vi "set_distance.vi"(3 "细分":u16=40000, 4 "速度(r/min)":u16, 5 "移动距离(mm)":dbl=1.0 caption="元素") -> (0 "指令":string, 1 "圈数":i32, 2 "脉冲数":i32)   [LabVIEW 2018]
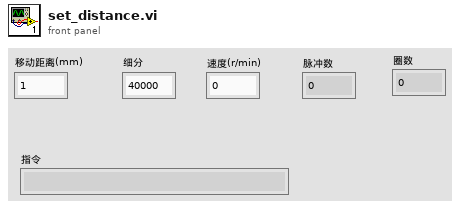
[diagram p1: front panel]
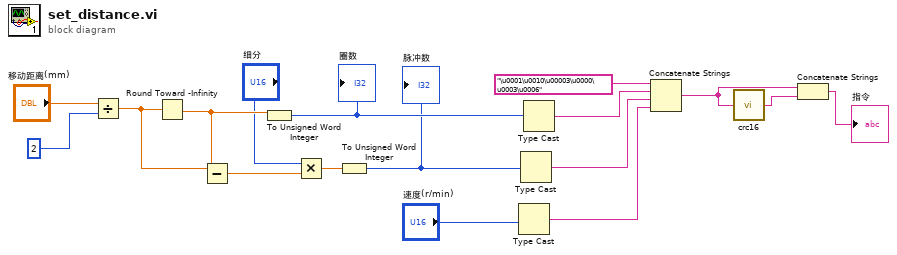
[diagram p0: block diagram]
diagram:
  n1 = Divide(x="移动距离(mm)", y=2) -> (x/y=w11:dbl)
  n2 = Round Toward -Infinity(1:w11) -> (0:w10:dbl)
  n3 = Subtract(x=w11, y=w10) -> (x-y=w9:dbl)
  n4 = To Unsigned Word Integer(number=w10) -> (unsigned 16bit integer=w5:u16)
  "圈数" <- w5
  n5 = Multiply(x="细分", y=w9) -> (x*y=w7:dbl)
  n6 = To Unsigned Word Integer(number=w7) -> (unsigned 16bit integer=w4:u16)
  "脉冲数" <- w4
  n7 = Type Cast(x="速度(r/min)") -> (*(type *) &x=w1:string)  [unwired: 1 in]
  n8 = Type Cast(x=w4) -> (*(type *) &x=w3:string)  [unwired: 1 in]
  n9 = Type Cast(x=w5) -> (*(type *) &x=w16:string)  [unwired: 1 in]
  n10 = Concatenate Strings("\u0001\u0010\u00003\u0000\u0003\u0006" ("字符串"), w16, w3, w1) -> (w17:string)
  n11 = call "crc16.vi"("message"=w17) -> ("CRC16"=w15:string)  [unwired: 4 in]
  n12 = Concatenate Strings(w17, w15) -> (→"指令":string)
